vi "PSDATA_Variant To I32.vi"(9 "error in":errorcluster, 10 "Value":variant) -> (1 "error out":errorcluster, 2 "Value":string, 4 "I32":i32)   [LabVIEW 2016]
doc: "Developer：YDX"
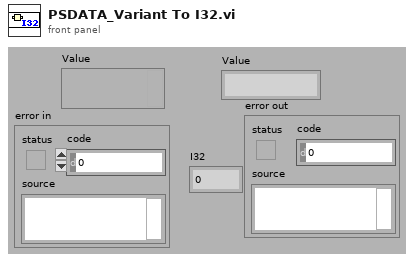
[diagram p1: front panel]
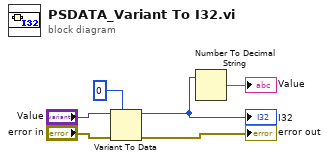
[diagram p0: block diagram]
diagram:
  n1 = Variant To Data(error in="error in", type=0 ("Str"), Variant="Value") -> (data=w1:i32, error out=→"error out":errorcluster)
  "I32" <- w1
  n2 = Number To Decimal String(number=w1) -> (decimal integer string=→"Value":string)  [unwired: 1 in]
